vi "Initialize.vi"(5 "Prepend Result Name":bool, 6 "Folder Path":path, 7 "Include All Evaluations?":bool, 8 "Error In":errorcluster, 9 "Active Sequence File":refnum<k7>, 10 "Engine Reference":refnum<k7>, 11 "Measurement Interface In":refnum<class "Measurement Interface.lvclass">) -> (0 "Error Out":errorcluster, 3 "Measurement Interface out":refnum<class "Measurement Interface.lvclass">)   [LabVIEW 2016, in "Measurement Interface.lvlib" / "Measurement Interface.lvclass"]
uses:
  Measurement Interface.lvclass
  Measurement Interface.lvclass/Measurement Interface.ctl
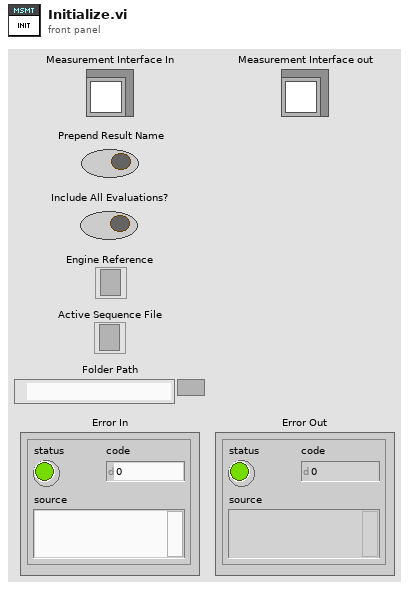
[diagram p1: front panel]
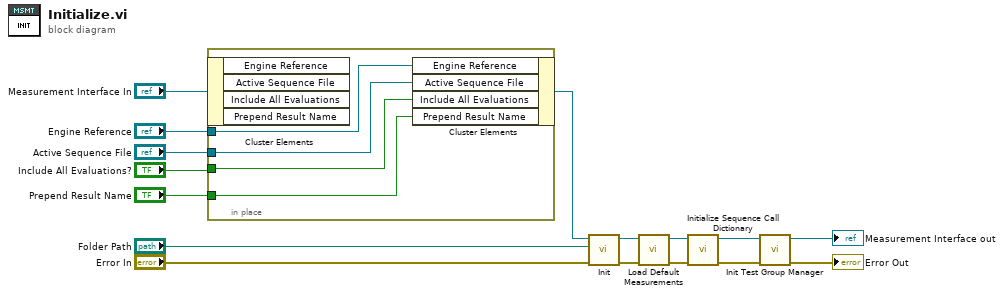
[diagram p0: block diagram]
diagram:
  n1 = in-place {
    in-place-border: "Engine Reference" -> [w20]
    in-place-border: "Active Sequence File" -> [w19]
    in-place-border: "Include All Evaluations?" -> [w18]
    in-place-border: "Prepend Result Name" -> [w17]
    n2 = in-place-cluster #1("Measurement Interface In") -> ()  [unwired: 4 out]
    n3 = in-place-cluster #1("Engine Reference"=w20, "Active Sequence File"=w19, "Include All Evaluations"=w18, "Prepend Result Name"=w17) -> (w13:refnum<class "Measurement Interface.lvclass">)
  }
  n4 = call-dynamic "Init.vi"("Error In"="Error In", "Folder Path"="Folder Path", "Plugin Framework In"=w13) -> ("Error Out"=w15:errorcluster, "Measurement Interface out"=w8:refnum<class "Measurement Interface.lvclass">)  [unwired: 7 in]
  n5 = call "Load Default Measurements.vi"("error in (no error)"=w15, "Measurement Interface in"=w8) -> ("error out"=w9:errorcluster, "Measurement Interface out"=w6:refnum<class "Measurement Interface.lvclass">)  [unwired: 8 in]
  n6 = call "Initialize Sequence Call Dictionary.vi"("error in (no error)"=w9, "Measurement Interface in"=w6) -> ("error out"=w7:errorcluster, "Measurement Interface out"=w4:refnum<class "Measurement Interface.lvclass">)  [unwired: 8 in]
  n7 = call "Init Test Group Manager.vi"("error in (no error)"=w7, "Measurement Interface in"=w4) -> ("error out"=→"Error Out":errorcluster, "Measurement Interface out"=→"Measurement Interface out":refnum<class "Measurement Interface.lvclass">)  [unwired: 8 in]
